vi "Main.vi"() -> ()   [LabVIEW 2017]
doc: "The myRIO Project template acquires acceleration data from the onboard accelerometer and displays the changes of acceleration values in a waveform chart."
uses:
  <vilib>/myRIO/Express VI/Onboard IO/PWM/PWM Express VI.xnode
  <vilib>/myRIO/Instrument Drivers/Onboard IO/PWM/vis/Set Duty Cycle and Frequency.vi
  <vilib>/myRIO/Instrument Drivers/Onboard IO/PWM/typedefs/PWM Configuration.ctl
  <vilib>/myRIO/Common/Instrument Driver Framework/myRIO v1.0/PWM/typedefs/PWM Channels Enum.ctl
  <vilib>/myRIO/Common/Instrument Driver Framework/Utilities/typedefs/Generic FPGA Reference.ctl
  <vilib>/myRIO/Common/Instrument Driver Framework/Utilities/typedefs/myRIO v1.0 Reference.ctl
  <vilib>/myRIO/Common/Instrument Driver Framework/Utilities/typedefs/Hardware Version Enum.ctl
  <vilib>/myRIO/Common/Instrument Driver Framework/Utilities/typedefs/myRIO Generic Hardware Reference.ctl
  <vilib>/myRIO/Instrument Drivers/Onboard IO/PWM/typedefs/PWM Reference.ctl
  <vilib>/myRIO/Instrument Drivers/Onboard IO/PWM/vis/myRIO PWM Open.xnode
  <vilib>/myRIO/Common/Instrument Driver Framework/Utilities/vis/Is FPGA Ref Available.vi
  <vilib>/myRIO/Common/Instrument Driver Framework/myRIO v1.0/PWM/vis/myRIO v1.1 Open PWM.vi
  <vilib>/userdefined/High Color/nirio_resource_hc.ctl
panel:
  out "Numeric Control":i32
  in  "X Axis":T1
  in  "Y Axis":cluster{"Frequency":dbl, "FWD/RVS":bool}
  in  "stop":bool
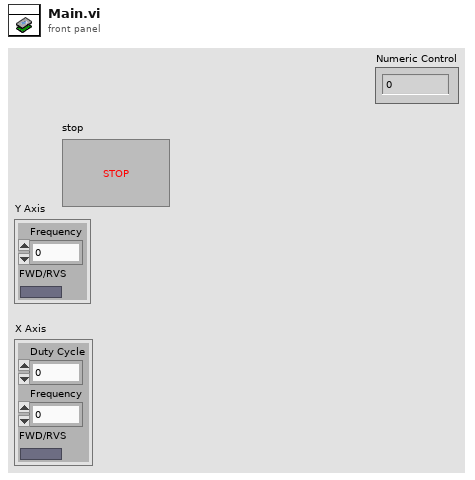
[diagram p1: front panel]
types:
  T1 = cluster{"Duty Cycle":dbl, "Frequency":dbl, "FWD/RVS":bool}
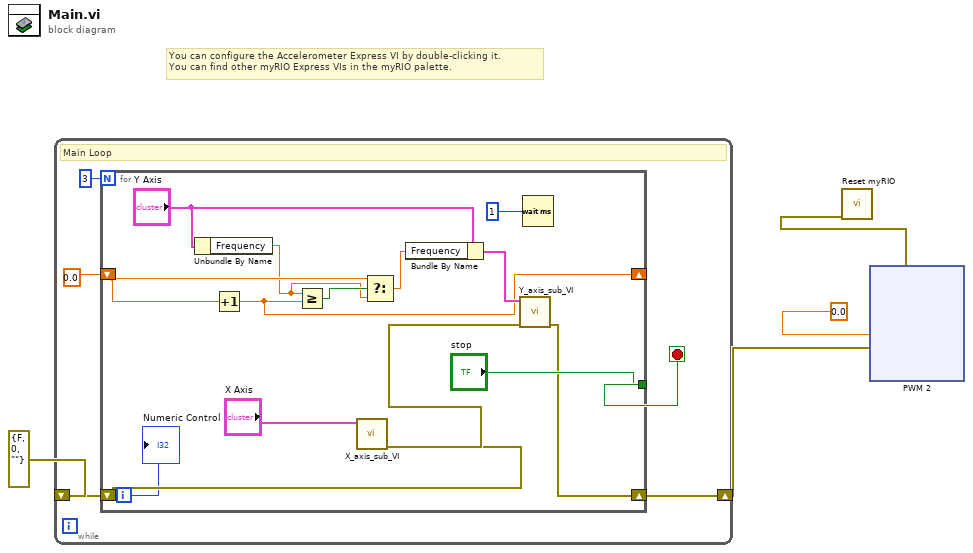
[diagram p0: block diagram]
diagram:
  # "You can configure the Accelerometer Express VI by double-clicking it.\nYou can find other myRIO Express VIs in the myRIO palette."
  n1 = while {
    shift-right: [w7] -> w3
    shift-left: errorcluster {"status"=FALSE, "code"=0, "source"=""} ("error in (no error)") -> [w9]
    stop <- w8 stop-if-true
    # "Main Loop"
    n2 = for {
      N: 3 -> [_]
      tunnel: ["stop"] -> w8
      shift-right: [w16] -> w7
      shift-left: w9 -> [w21]
      shift-right: [w11] -> _
      shift-left: 0.0 -> [w13]
      i -> [w10]
      n3 = Unbundle By Name("Y Axis") -> ("Frequency"=w12:dbl)
      n4 = Increment(x=w13) -> (x+1=w11:dbl)
      n5 = Greater Or Equal?(x=w12, y=w11) -> (x >= y?=w14:bool)
      n6 = call "X_axis_sub_VI.vi"("error in (no error)"=w21, "X Axis"="X Axis") -> ("error out"=w22:errorcluster)  [unwired: 9 in]
      n7 = Select(t=w13, s=w14, f=w12) -> (s? t:f=w15:dbl)
      n8 = Bundle By Name(cluster="Y Axis", "Frequency"=w15) -> (w18:cluster{"Frequency":dbl, "FWD/RVS":bool})
      n9 = call "Y_axis_sub_VI.vi"("error in (no error)"=w22, "Y Axis"=w18) -> ("error out"=w16:errorcluster)  [unwired: 9 in]
      n10 = Wait (ms)(milliseconds to wait=u32 1) -> ()  [unwired: 1 out]
      "Numeric Control" <- w10
    }
  }
  n11 = xnode "PWM 2"("Frequency [Hz]"=0.0, "error in (no error)"=w3) -> ("error out"=w2:errorcluster)
  n12 = call <vilib>:"Reset myRIO.vi"("error in (no error)"=w2) -> ()  [unwired: 10 in, 1 out]
